vi "ProdaNG.TestStepParam.New.vi"(8 "error in (no error)":errorcluster, 10 "TestStepParam":T1 {"value" format="%#.3f"}, 11 "dbHandleIn":i32) -> (0 "error out":errorcluster, 2 "TestStepParam out":T1 {"value" format="%#.3f"}, 3 "dbHandle":i32)   [LabVIEW 2016]
doc: "This function returns a product structure for a product, which is identified by a part and a serial number.\nImportant information: The field 'individual' was taken over from the field 'allgemein' of the legacy data directly. Because of this most products have the value 0 further on and only a few the value 1. \nParameter:\nhandle is an Integer, which is returned by the function Login() at the creation of a new connection.\nwabcoPartId is the Id of the part.\nserialNumber is the serial number of the product for the part above.\nproduct is a pointer on a product structure, which is filled if the returncode is 0. The structure must be defined in the calling program.\n\nReturncodes:\n0 No error\n< 0 ORACLE Error code\n6 (ERROR_INVALID_HANDLE) in case of an invalid handle\n1403 Record does not exist"
uses:
  Controls/ProdaNG.TestStepParam.ctl
  Controls/ProdaNG.TestStepParamSize.ctl
  prodllNG.dll
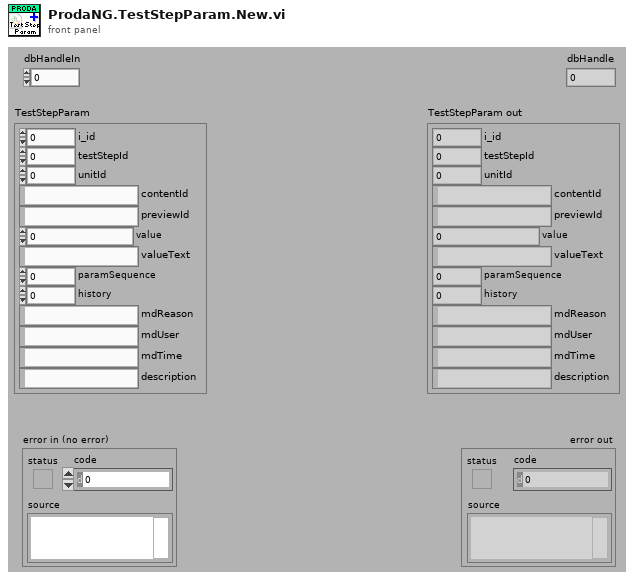
[diagram p1: front panel]
types:
  T1 = typedef "ProdaNG.TestStepParam.ctl" = cluster{"i_id":i32, "testStepId":i32, "unitId":i32, "contentId":string, "previewId":string, "value":dbl, "valueText":string, "paramSequence":i32, "history":i32, "mdReason":string, "mdUser":string, "mdTime":string, "description":string}
  T2 = typedef "ProdaNG.TestStepParamSize.ctl" = cluster{"i_id":i32, "testStepId":i32, "unitId":i32, "contentId":i32, "previewId":i32, "value":i32, "valueText":i32, "paramSequence":i32, "history":i32, "mdReason":i32, "mdUser":i32, "mdTime":i32, "description":i32}
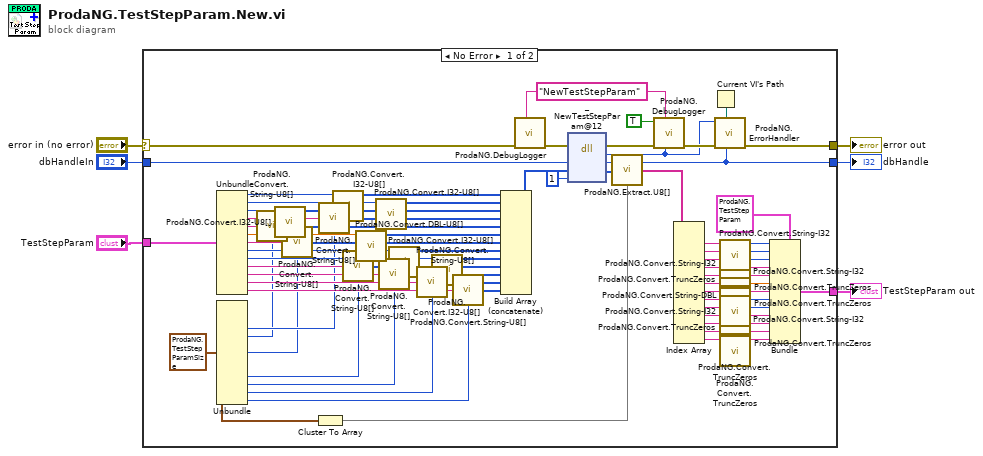
[diagram p0: block diagram]
diagram:
  n1 = case shown="No Error" "error in (no error)" {
    selector: "error in (no error)" -> [w80 w87]
    tunnel: [w85 w87] -> w5
    tunnel: "dbHandleIn" -> [w82 w86]
    tunnel: [w83 w86] -> w3
    tunnel: "TestStepParam" -> [w10 _]
    tunnel: [w47 _] -> w1
    frame No Error {
      w11 = T2 {"i_id"=4, "testStepId"=4, "unitId"=4, "contentId"=16, "previewId"=16, "value"=8, "valueText"=258, "paramSequence"=4, "history"=4, "mdReason"=514, "mdUser"=22, "mdTime"=24, "description"=514} ("TestStepSize")
      w76 = "NewTestStepParam" ("cmd")
      n2 = Unbundle(w10) -> ("i_id"=w40:i32, "testStepId"=w43:i32, "unitId"=w38:i32, "contentId"=w42:string, "previewId"=w35:string, "value"=w36:dbl, "valueText"=w20:string, "paramSequence"=w18:i32, "history"=w17:i32, "mdReason"=w32:string, "mdUser"=w31:string, "mdTime"=w30:string, "description"=w29:string)
      n3 = Unbundle(w11) -> ("contentId"=w14:i32, "previewId"=w13:i32, "valueText"=w12:i32, "mdReason"=w24:i32, "mdUser"=w23:i32, "mdTime"=w22:i32, "description"=w21:i32)  [unwired: 6 out]
      n4 = call "ProdaNG.Convert.String-U8[].vi"("Input String"=w35, "Size"=w13) -> ("Output"=w34:u8[])
      n5 = call "ProdaNG.Convert.I32-U8[].vi"("32bit integer"=w38) -> ("unsigned byte array"=w37:u8[])  [unwired: 10 in]
      n6 = call "ProdaNG.Convert.String-U8[].vi"("Input String"=w20, "Size"=w12) -> ("Output"=w19:u8[])
      n7 = Cluster To Array(cluster=w11) -> (array=w8:i32[])
      n8 = call "ProdaNG.Convert.String-U8[].vi"("Input String"=w42, "Size"=w14) -> ("Output"=w41:u8[])
      n9 = call "ProdaNG.Convert.I32-U8[].vi"("32bit integer"=w40) -> ("unsigned byte array"=w39:u8[])  [unwired: 10 in]
      n10 = call "ProdaNG.Convert.String-U8[].vi"("Input String"=w32, "Size"=w24) -> ("Output"=w25:u8[])
      n11 = call "ProdaNG.Convert.DBL-U8[].vi"("dbl"=w36) -> ("unsigned byte array"=w33:u8[])  [unwired: 10 in]
      n12 = call "ProdaNG.Convert.I32-U8[].vi"("32bit integer"=w43) -> ("unsigned byte array"=w44:u8[])  [unwired: 10 in]
      n13 = call "ProdaNG.Convert.String-U8[].vi"("Input String"=w31, "Size"=w23) -> ("Output"=w26:u8[])
      n14 = call "ProdaNG.Convert.I32-U8[].vi"("32bit integer"=w18) -> ("unsigned byte array"=w16:u8[])  [unwired: 10 in]
      n15 = call "ProdaNG.Convert.String-U8[].vi"("Input String"=w30, "Size"=w22) -> ("Output"=w27:u8[])
      n16 = call "ProdaNG.Convert.I32-U8[].vi"("32bit integer"=w17) -> ("unsigned byte array"=w15:u8[])  [unwired: 10 in]
      n17 = call "ProdaNG.Convert.String-U8[].vi"("Input String"=w29, "Size"=w21) -> ("Output"=w28:u8[])
      n18 = Build Array (concatenate)(w39, w44, w37, w41, w34, w33, w19, w16, w15, w25, w26, w27, w28) -> (w9:u8[])
      n19 = call "ProdaNG.DebugLogger.vi"("cmd"=w76, "error in (no error)"=w80) -> ("error out"=w79:errorcluster)  [unwired: 9 in]
      n20 = dll-call lib="D:/Maszup/WABCO/SVN/LineTraceSystem/SOFTWARE/sources/Database/ProdaNG/prodllNG.dll" fn="_NewTestStepParam@12" ("ProDLL wrapper.dll:ProDLL_wrapper_GetWabcoParts_GetData")(error in=w79, "dbHandle"=w82, "testStepParams"=w9, "doCommit"=1) -> (error out=w78:errorcluster, "return type"=w75:i32, "dbHandle"=w83:i32, "testStepParams"=w45:u8[])  [unwired: 3 in, 1 out]
      n21 = call "ProdaNG.Extract.U8[].vi"("unsigned byte array"=w45, "Sizes"=w8) -> ("Elements"=w7:string[])
      n22 = call "ProdaNG.DebugLogger.vi"("return type"=w75, "cmd"=w76, "error in (no error)"=w78, "done? (F)"=TRUE) -> ("error out"=w77:errorcluster)  [unwired: 7 in]
      n23 = Index Array(array=w7) -> (element #1=w74:string, element #2=w71:string, element #3=w70:string, element #4=w54:string, element #5=w51:string, element #6=w50:string, element #7=w55:string, element #8=w66:string, element #9=w65:string, element #10=w57:string, element #11=w58:string, element #12=w59:string, element #13=w60:string)  [unwired: 13 in]
      n24 = Current VI's Path() -> (path=w84:path)
      n25 = call "ProdaNG.ErrorHandler.vi"("dbHandleIn"=w83, "Path"=w84, "error in"=w77, "output_parameter"=w75) -> ("error out"=w85:errorcluster)  [unwired: 7 in]
      n26 = call "ProdaNG.Convert.String-I32.vi"("unsigned byte string"=w74) -> ("32bit integer"=w73:i32)  [unwired: 10 in]
      n27 = call "ProdaNG.Convert.String-I32.vi"("unsigned byte string"=w71) -> ("32bit integer"=w72:i32)  [unwired: 10 in]
      n28 = call "ProdaNG.Convert.String-I32.vi"("unsigned byte string"=w70) -> ("32bit integer"=w69:i32)  [unwired: 10 in]
      n29 = call "ProdaNG.Convert.TruncZeros.vi"("string with \\0s"=w54) -> ("LV string"=w53:string)  [unwired: 10 in]
      n30 = call "ProdaNG.Convert.TruncZeros.vi"("string with \\0s"=w51) -> ("LV string"=w52:string)  [unwired: 10 in]
      n31 = call "ProdaNG.Convert.String-DBL.vi"("unsigned byte string"=w50) -> ("dbl integer"=w49:dbl)  [unwired: 10 in]
      n32 = call "ProdaNG.Convert.TruncZeros.vi"("string with \\0s"=w55) -> ("LV string"=w56:string)  [unwired: 10 in]
      n33 = call "ProdaNG.Convert.String-I32.vi"("unsigned byte string"=w66) -> ("32bit integer"=w68:i32)  [unwired: 10 in]
      n34 = call "ProdaNG.Convert.String-I32.vi"("unsigned byte string"=w65) -> ("32bit integer"=w67:i32)  [unwired: 10 in]
      n35 = call "ProdaNG.Convert.TruncZeros.vi"("string with \\0s"=w57) -> ("LV string"=w63:string)  [unwired: 10 in]
      n36 = call "ProdaNG.Convert.TruncZeros.vi"("string with \\0s"=w58) -> ("LV string"=w64:string)  [unwired: 10 in]
      n37 = call "ProdaNG.Convert.TruncZeros.vi"("string with \\0s"=w59) -> ("LV string"=w62:string)  [unwired: 10 in]
      n38 = call "ProdaNG.Convert.TruncZeros.vi"("string with \\0s"=w60) -> ("LV string"=w61:string)  [unwired: 10 in]
      n39 = Bundle(cluster=T1 {"i_id"=0, "testStepId"=0, "unitId"=0, "contentId"="", "previewId"="", "value"=0.0, "valueText"="", "paramSequence"=0, "history"=0, "mdReason"="", "mdUser"="", "mdTime"="", "description"=""} ("TestStepParam out"), "i_id"=w73, "testStepId"=w72, "unitId"=w69, "contentId"=w53, "previewId"=w52, "value"=w49, "valueText"=w56, "paramSequence"=w68, "history"=w67, "mdReason"=w63, "mdUser"=w64, "mdTime"=w62, "description"=w61) -> (w47:T1)
    }
    frame Error {
    }
  }
  "error out" <- w5
  "dbHandle" <- w3
  "TestStepParam out" <- w1
